vi "Get Device Property (1D I32).vi"(0 "session in":refnum<k21>, 5 "devices":refnum<k21>="$DefaultDevices", 7 "property":refnum<k21>, 11 "error in (no error)":errorcluster) -> (4 "session out":refnum<k21>, 10 "property value":i32[](array[numeric]), 15 "error out":errorcluster)   [LabVIEW 2020, in "SLSC.lvlib"]
doc: "Gets the value of the specified device property from one or more devices."
uses:
  <vilib>/SLSC/SLSC.lvlib
  nislsclvapi.dll
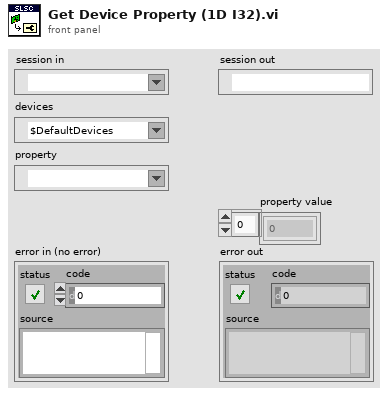
[diagram p1: front panel]
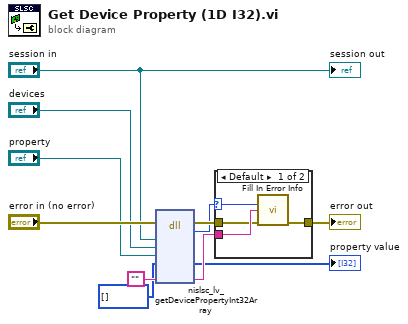
[diagram p0: block diagram]
diagram:
  n1 = dll-call lib="nislsclvapi.*" fn="nislsc_lv_getDevicePropertyInt32Array"(error in="error in (no error)", "session"="session in", "devices"="devices", "property"="property", "propertyValue"=i32[] [], "extendedErrorInfo"="") -> (error out=w8:errorcluster, w7:i32, "propertyValue"=→"property value":i32[], "extendedErrorInfo"=w9:string)  [unwired: 7 in, 1 out]
  n2 = case shown="Default" w7 {
    selector: w7 -> [w15 _]
    tunnel: w9 -> [w14 _]
    tunnel: w8 -> [w13 w16]
    tunnel: [w12 w16] -> w6
    frame Default {
      n3 = call <vilib>:"Fill In Error Info.vi"("status code"=w15, "extended error info"=w14, "error in"=w13) -> ("error out"=w12:errorcluster)  [unwired: 12 in]
    }
    frame 0 {
    }
  }
  "error out" <- w6
  "session out" <- "session in"
